vi "VNA_sweepCenterfreq.vi"(4 "Fc Start (Hz)":dbl=500000000.0 format="%#_6p", 7 "VNA Address":refnum<visa-resource-name>="GPIB0::15::INSTR", 11 "Transport":refnum<class "Transport.lvclass">=refnum) -> ()   [LabVIEW 2019]
uses:
  <userlib>/LevyLab/Transport/Transport/Transport.lvclass
  <userlib>/LevyLab/Transport/Control Experiment/Control Experiment.lvclass
  <userlib>/LevyLab/Lockin-Multichannel/Instrument.Lockin/Instrument.Lockin.lvclass
  <userlib>/LevyLab/Instrument Framework/subsystems/API/API.lvclass
  <userlib>/LevyLab/Configuration/Configuration.lvclass
  <userlib>/LevyLab/Instrument Framework/subsystems/HAL/HAL.lvclass
  <userlib>/LevyLab/Logger.PGSQL/Logger.PGSQL/Logger.PGSQL.lvclass
  <userlib>/LevyLab/Logger.Error/Logger.Error/Logger.Error.lvclass
  <userlib>/LevyLab/RemoteControl/RemoteControl/RemoteControl.lvclass
  <userlib>/LevyLab/Lockin-Multichannel/Instrument.DAQ/Instrument.DAQ.lvclass
  <userlib>/LevyLab/Krohn Hite 7008/Inst.Krohn-Hite-7008/Inst.Krohn-Hite-7008.lvclass
  <userlib>/LevyLab/Leiden API/Inst.TC.MNK/Inst.TC.MNK.lvclass
  <userlib>/LevyLab/Leiden API/FP-TC-Shared/FP-TC-Shared.lvclass
  <userlib>/LevyLab/Oxford-1820/Instrument.Oxford1820/Instrument.Oxford1820.lvclass
  <userlib>/LevyLab/RemoteControl.ZMQ/RemoteControl.ZMQ/RemoteControl.ZMQ.lvclass
  <vilib>/addons/zeromq/zmq_socket.lvclass
  <userlib>/LevyLab/Instrument Framework/Instrument Types/Cryostat/Instrument.Cryostat.lvclass
  <userlib>/LevyLab/Instrument Framework/Instrument Types/CBridge/Instrument.CBridge.lvclass
  <userlib>/LevyLab/Instrument Framework/Instrument Types/Delay Line/Instrument.DelayLine.lvclass
  <userlib>/LevyLab/Instrument Framework/Instrument Types/Strain/Instrument.Strain.lvclass
  <userlib>/LevyLab/Instrument Framework/Instrument Types/VNA/Instrument.VNA.lvclass
  <userlib>/LevyLab/Instrument Framework/Instrument Types/VSource/Instrument.VSource.lvclass
  <userlib>/LevyLab/Transport/Transport/Transport.lvclass/Transport.ctl
  <userlib>/LevyLab/Transport/Control Experiment/Control Experiment.lvclass/Control Experiment.ctl
  <instrlib>/Agilent 87XX Series/Agilent 87XX Series.lvlib
panel:
  in  "Experiment Folder 2":string="06-test"
  in  "Experiment Description 2":string="T<30mK\nVbg(AO4) = 0V\nB=changing\nPower: -32 dBm\nVd: 1.3V\nId: 9.55mA \nBW = 300 Hz \nAvg =1\n"
  in  "Fc Step (Hz)":dbl=500000000.0 format="%#_6p"
  in  "Fc End (Hz)":dbl=1000000000.0 format="%#_6p"
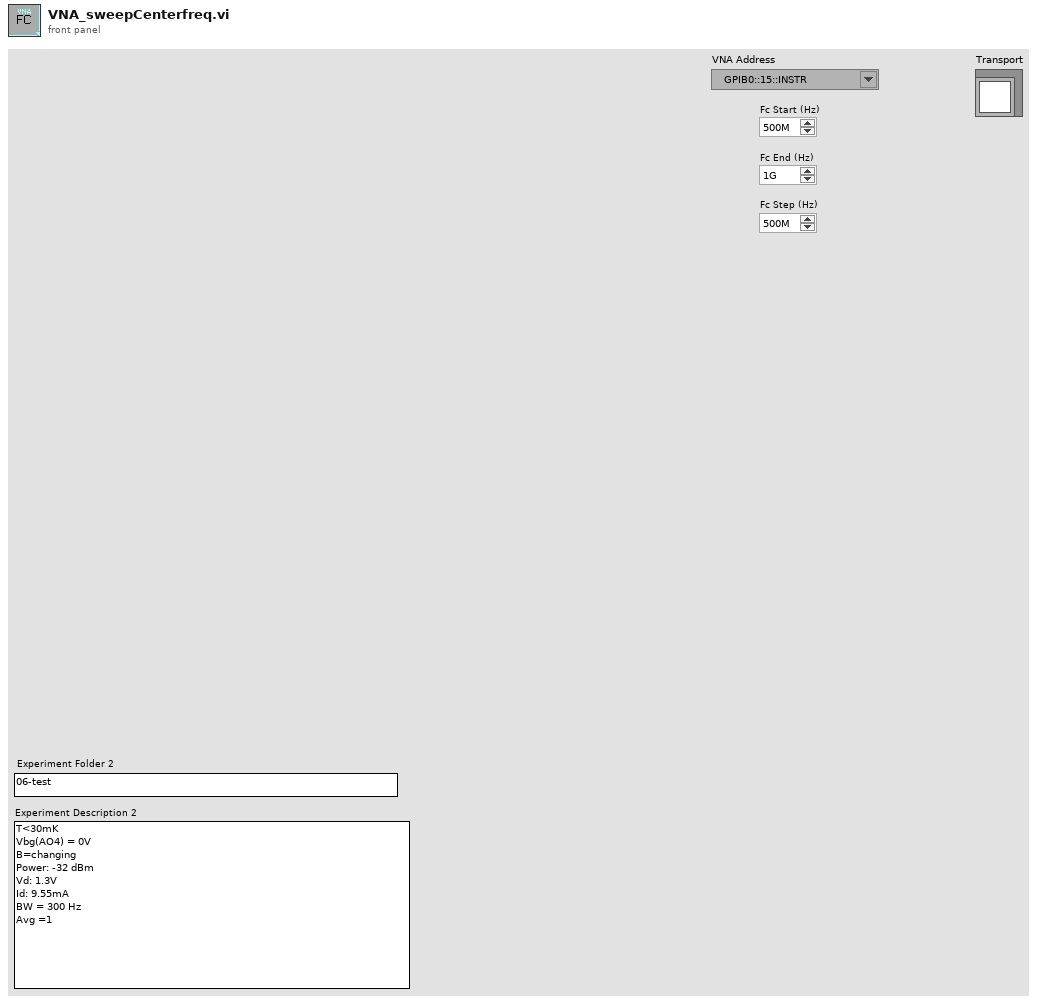
[diagram p1: front panel]
types:
  T1 = enum32{"Bad", "Idle", "Run top level", "Running"}
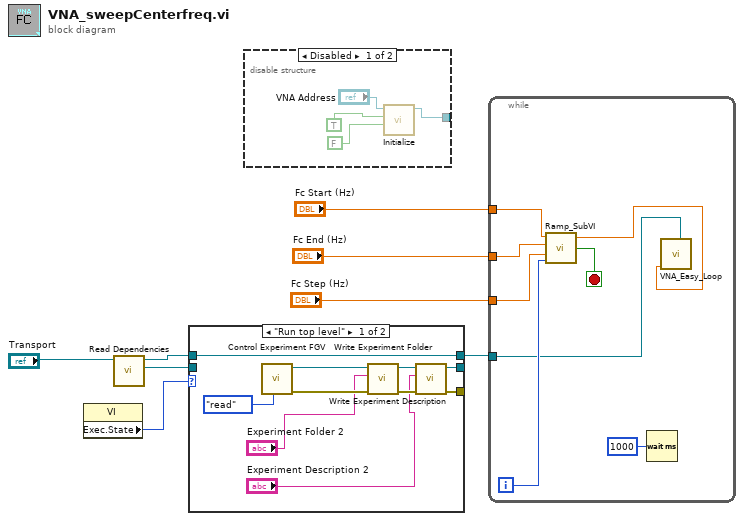
[diagram p0: block diagram]
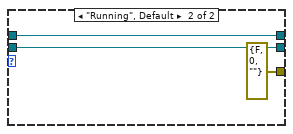
[diagram p2: hidden frame]
diagram:
  n1 = property class="VI"() -> ("Exec.State"=w5:T1)  [unwired: 2 in, 2 out]
  n2 = call <userlib>:"Read Dependencies.vi"("Transport"="Transport") -> ("C.E."=w4:refnum<class "Control Experiment.lvclass">, "Transport"=w3:refnum<class "Transport.lvclass">)  [unwired: 8 in, 1 out]
  n3 = case shown="\"Run top level\"" w5 {
    tunnel: [w14 errorcluster {"status"=FALSE, "code"=0, "source"=""} ("error out")] -> _
    tunnel: [w13 w21] -> _
    tunnel: w4 -> [_ w21]
    tunnel: w3 -> [w9 w19]
    tunnel: [w9 w19] -> w2
    frame "Run top level" {
      n4 = call <userlib>:"Control Experiment FGV.vi"("Function"=enum16{"read", "write"}."read") -> ("error out"=w17:errorcluster, "Control Experiment.lvclass out"=w18:refnum<class "Control Experiment.lvclass">)  [unwired: 9 in]
      n5 = call <userlib>:"Write Experiment Folder.vi"("error in (no error)"=w17, "Experiment Folder"="Experiment Folder 2", "Control Experiment in"=w18) -> ("error out"=w15:errorcluster, "Control Experiment out"=w16:refnum<class "Control Experiment.lvclass">)  [unwired: 7 in]
      n6 = call <userlib>:"Write Experiment Description.vi"("error in (no error)"=w15, "Experiment Description"="Experiment Description 2", "Control Experiment in"=w16) -> ("error out"=w14:errorcluster, "Control Experiment out"=w13:refnum<class "Control Experiment.lvclass">)  [unwired: 7 in]
    }
    frame "Running", Default {
    }
  }
  n7 = disable-structure shown="Disabled" {
    disable-tunnel: [w22 _] -> _
    frame Disabled {
      n8 = call <instrlib>:"Initialize.vi"("reset"=FALSE, "ID query"=TRUE, "VISA resource name"="VNA Address") -> ("VISA resource name out"=w22:refnum<visa-resource-name>)  [unwired: 7 in, 1 out]
    }
    frame Enabled {
    }
  }
  n9 = while {
    tunnel: "Fc Start (Hz)" -> [w33]
    tunnel: "Fc End (Hz)" -> [w32]
    tunnel: "Fc Step (Hz)" -> [w31]
    tunnel: w2 -> [w27]
    i -> [w30]
    stop <- w29 stop-if-true
    n10 = call <userlib>:"Ramp_SubVI.vi"("index"=w30, "step"=w31, "end"=w32, "start"=w33) -> ("Stop?"=w29:bool, "Numeric"=w26:dbl)  [unwired: 1 in]
    n11 = Wait (ms)(milliseconds to wait=u32 1000) -> ()  [unwired: 1 out]
    n12 = call "VNA_Easy_Loop.vi"("Transport"=w27, "start/center"=w26) -> ()  [unwired: 8 in, 2 out]
  }
